vi "FPGA Main Image Processing.vi"(9 "?":T1) -> ()   [LabVIEW 2025]
doc: "The myRIO v1.1 FPGA Shipping Personality. This personality contains support for:\n- 2 Analog Input Interrupt channel\n- 4 Digital Input Interrupt channel\n- 1 Timer\n- 1 Accelerometer\n- 1 Button\n- 4 LED\n- 10 Analog Input channels with 1 Sample\n- 6 Analog Output channels with 1 Sample\n- 40 Digital I/O channels with 1 Sample\n- 2 I2C channels\n- 4 Encoder channels\n- 6 PWM channels\n- 2 SPI channels"
uses:
  SoC IP Library/Controls/Ocurrences.ctl
  SoC IP Library/Controls/Image Size.ctl
  <vilib>/rvi/Emulation/niFpgaGetClockAttributes.vi
  <vilib>/rvi/Emulation/niFpgaSctlEmulationGetInTimedLoop.vi
  <vilib>/rvi/Emulation/niFpgaEmulationReportErrorSimple.vi
  <vilib>/rvi/Emulation/niFpgaProcessEmulError.vi
  <vilib>/rvi/DataTransferAndStorage/Container/Common/niFpgaContainerGetUniqueNameForEmu.vi
  <vilib>/rvi/DataTransferAndStorage/Container/Common/niFpgaContainerSetEmuInfo.vi
  <vilib>/rvi/eio/common/nirviEmuReportErrorAndStop.vi
  <vilib>/rvi/Memory/Memory_Emulation/nirvimemoryFastEmulation.vi
  <vilib>/rvi/Memory/Memory_Emulation/nirvimemoryEmulation.vi
  <vilib>/rvi/Emulation/niFpgaEmulationIsFPGAContextNoSignature.vi
  <vilib>/rvi/errors/nirviReportUnexpectedCaseInternalError (U32).vi
  <vilib>/eio/utilities/niEioResolveVilibRelativePath.vi
  <vilib>/rvi/interface/RandomDataEmulation/niFpgaRandomDataHandleErrors.vi
  <vilib>/rvi/Emulation/niFpgaCriticalErrorInLSC.vi
  <vilib>/rvi/LocalResourceManager/LocalResourceManager.xnode
  <vilib>/rvi/DataTransferAndStorage/Container/XNode/niFpgaContainer.xnode
  <vilib>/rvi/interface/RandomDataEmulation/nirviRandomDataFpgaReadWriteTemplate.vi
  <vilib>/rvi/FXPMathLib/basic elements/FxpDiscreteDelay/XNode/nifxpmath_DiscreteDelay.xnode
  SoC IP Library/SoC IP Library.lvlib
panel:
  out "Current Colum Process":u8
  out "Current Row Process":u8
  out "Current Colum Write":u8
  out "Current Row Write":u8
  out "Current Colum Read":u8
  out "Current Row Read":u8
  out "Pixel B Write":u16
  out "Pixel A Write":u16
  out "SYS.OCURRENCES.RDY":bool
  out "SYS.IMG_SIZE.RDY":bool
  out "Image size":u32
  out "SYS.RDY":bool
  # "Image Processing"
  # "System"
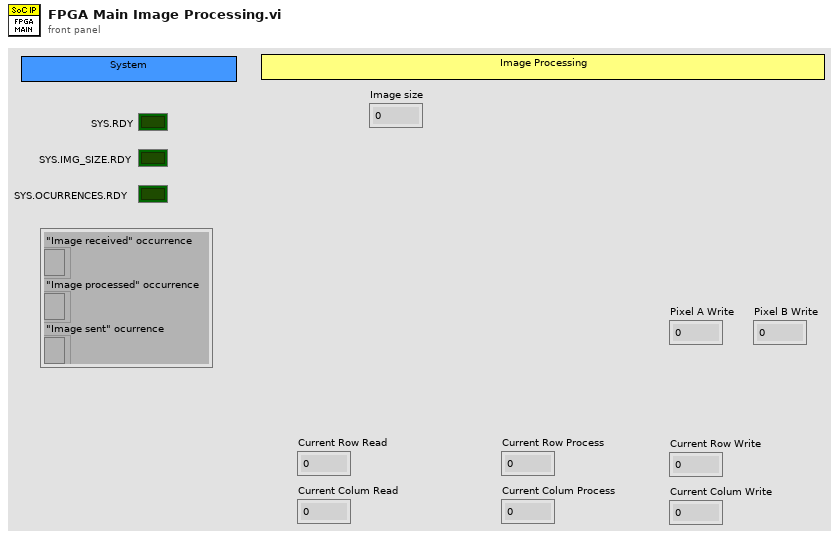
[diagram p1: front panel]
types:
  T1 = typedef "SoC IP Library.lvlib/Ocurrences.ctl" = cluster{"\"Image received\" occurrence":refnum<k4>, "\"Image processed\" occurrence":refnum<k4>, "\"Image sent\" ocurrence":refnum<k4>}
  T2 = typedef "SoC IP Library.lvlib/Image Size.ctl" = cluster{"Rows (X)":u16, "Colums (Y)":u16}
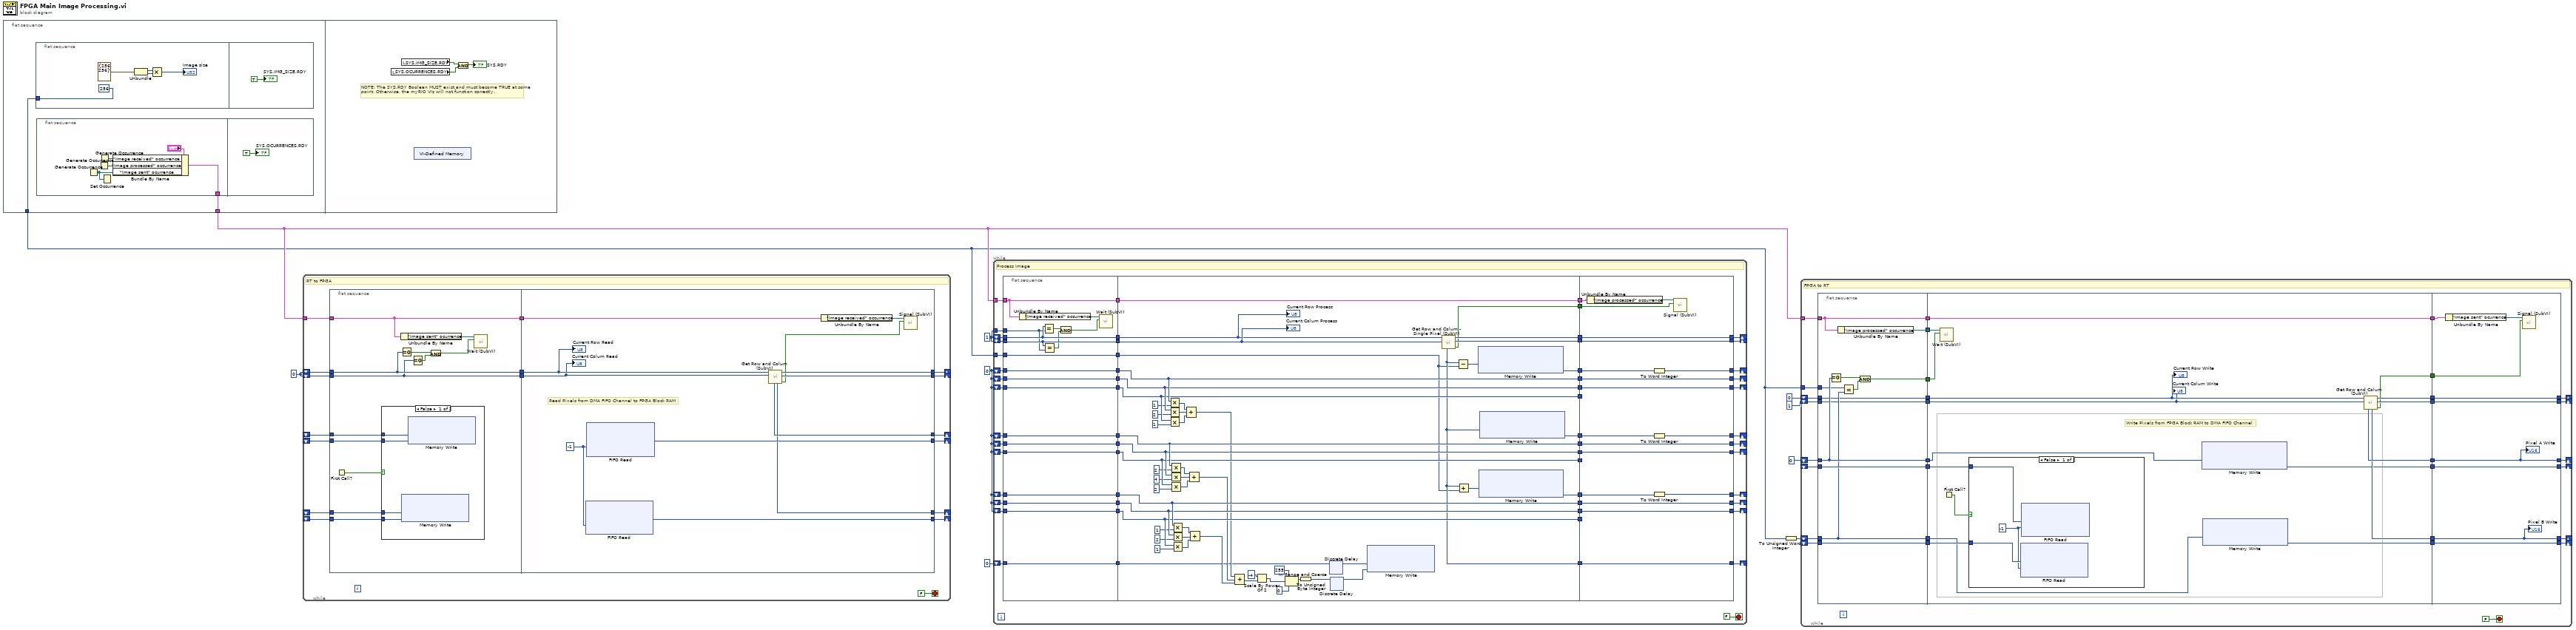
[diagram p0: block diagram]
diagram:
  w2 = i16 0 ("Data")
  w3 = u8 1 ("Row Out")
  w8 = u8 0
  n1 = flat-sequence {
    tunnel: [w12] -> w5
    tunnel: [w11] -> w6
    frame #0 {
      n2 = flat-sequence {
        tunnel: [u32 256 ("Dimension")] -> w12
        frame #0 {
          n3 = Unbundle(T2 {"Rows (X)"=256, "Colums (Y)"=256} ("Image Size")) -> ("Rows (X)"=w21:u16, "Colums (Y)"=w22:u16)
          n4 = Multiply(x=w21, y=w22) -> (x*y=→"Image size":u32)
        }
        frame #1 {
          "SYS.IMG_SIZE.RDY" <- TRUE
        }
      }
      n5 = flat-sequence {
        tunnel: [w13] -> w11
        frame #0 {
          n6 = Generate Occurrence() -> (w14:refnum<k4>)
          n7 = Generate Occurrence() -> (w15:refnum<k4>)
          n8 = Generate Occurrence() -> (w16:refnum<k4>)
          n9 = Set Occurrence(w14) -> ()
          n10 = Bundle By Name(cluster="?", "\"Image received\" occurrence"=w16, "\"Image processed\" occurrence"=w15, "\"Image sent\" ocurrence"=w14) -> (w13:T1)
        }
        frame #1 {
          "SYS.OCURRENCES.RDY" <- TRUE
        }
      }
    }
    frame #1 {
      # "NOTE: The SYS.RDY Boolean MUST exist and must become TRUE at some point. Otherwise, the myRIO VIs will not function correctly."
      n11 = local read "SYS.OCURRENCES.RDY"() -> (w26:bool)
      n12 = local read "SYS.IMG_SIZE.RDY"() -> (w25:bool)
      n13 = xnode "VI-Defined Memory"() -> ()  [unwired: 1 out]
      n14 = And(x=w25, y=w26) -> (x .and. y?=→"SYS.RDY":bool)
    }
  }
  n15 = while {
    shift-right: [w37] -> _
    shift-left: _ -> [w44]
    shift-right: [w31] -> _
    shift-left: _ -> [w43]
    shift-right: [w36] -> _
    shift-left: _ -> [w42]
    shift-right: [w40] -> _
    shift-left: _ -> [w41]
    shift-right: [w39] -> _
    shift-left: w8 -> [w35]
    shift-right: [w38] -> _
    shift-left: w8 -> [w34]
    tunnel: w6 -> [w30]
    stop <- FALSE stop-if-true
    # "RT to FPGA"
    n16 = flat-sequence {
      tunnel: w34 -> [w54]
      tunnel: w35 -> [w55]
      tunnel: w41 -> [w47]
      tunnel: w42 -> [w45]
      tunnel: w43 -> [w48]
      tunnel: w44 -> [w46]
      tunnel: [w55] -> w33
      tunnel: [w54] -> w32
      tunnel: w30 -> [w56]
      tunnel: [w56] -> w29
      tunnel: w33 -> [w68]
      tunnel: w32 -> [w67]
      tunnel: w29 -> [w64]
      tunnel: [w72] -> w31
      tunnel: [w71] -> w40
      tunnel: [w70] -> w39
      tunnel: [w69] -> w38
      tunnel: [w63] -> w37
      tunnel: [w62] -> w36
      frame #0 {
        n17 = First Call?() -> (First Call?: T/F=w49:bool)
        n18 = case shown="False" w49 {
          tunnel: w46 -> [w60 _]
          tunnel: w48 -> [w59 _]
          tunnel: w47 -> [w58 _]
          tunnel: w45 -> [w57 _]
          frame False {
            n19 = xnode ("Memory Write")("Address"=w57, "Data"=w58) -> ()  [unwired: 1 in, 1 out]
            n20 = xnode ("Memory Write")("Address"=w60, "Data"=w59) -> ()  [unwired: 1 in, 1 out]
          }
          frame True {
          }
        }
        n21 = Equal To 0?(x=w55) -> (x = 0?=w52:bool)
        n22 = Unbundle By Name(w56) -> ("\"Image sent\" ocurrence"=w51:refnum<k4>)
        n23 = Equal To 0?(x=w54) -> (x = 0?=w50:bool)
        n24 = And(x=w52, y=w50) -> (x .and. y?=w53:bool)
        n25 = call "Wait (SubVI).vi"("Wait? (T)"=w53, "Occurrence in"=w51) -> ()  [unwired: 10 in]
      }
      frame #1 {
        w65 = -1 ("Timeout")
        # "Read Pixels from DMA FIFO Channel to FPGA Block RAM"
        n26 = xnode ("FIFO Read")("Timeout"=w65) -> ("Element"=w71:u8)  [unwired: 1 in, 2 out]
        n27 = xnode ("FIFO Read")("Timeout"=w65) -> ("Element"=w72:u8)  [unwired: 1 in, 2 out]
        n28 = call "Get Row and Colum (SubVI).vi"("Colum In"=w67, "Row In"=w68) -> ("Last Pixel?"=w66:bool, "Colum Out"=w69:u8, "Row Out"=w70:u8, "Pixel B"=w62:u16, "Pixel A"=w63:u16)  [unwired: 5 in]
        n29 = Unbundle By Name(w64) -> ("\"Image received\" occurrence"=w61:refnum<k4>)
        n30 = call "Signal (SubVI).vi"("Set? (T)"=w66, "Occurrence in"=w61) -> ()  [unwired: 10 in]
        "Current Row Read" <- w68
        "Current Colum Read" <- w67
      }
    }
  }
  n31 = while {
    tunnel: w6 -> [w130]
    shift-right: [w126] -> _
    shift-left: w2 -> [w124]
    shift-right: [w122] -> _
    shift-left: w2 -> [w121]
    shift-right: [w118] -> _
    shift-left: w2 -> [w116]
    shift-right: [w113] -> _
    shift-left: w2 -> [w111]
    shift-right: [w109] -> _
    shift-left: w2 -> [w107]
    shift-right: [w105] -> _
    shift-left: w2 -> [w103]
    shift-right: [w100] -> _
    shift-left: w2 -> [w99]
    shift-right: [w96] -> _
    shift-left: w2 -> [w95]
    shift-right: [w92] -> _
    shift-left: w2 -> [w90]
    shift-right: [w87] -> _
    shift-left: w3 -> [w82]
    shift-right: [w85] -> _
    shift-left: w3 -> [w83]
    tunnel: w5 -> [w80]
    shift-right: [w76] -> _
    shift-left: u32 0 ("Pixel") -> [w78]
    tunnel: w3 -> [w74]
    stop <- FALSE stop-if-true
    # "Process Image"
    n32 = flat-sequence {
      tunnel: w130 -> [w149]
      tunnel: [w149] -> w128
      tunnel: [w148] -> w125
      tunnel: w124 -> [w148]
      tunnel: w121 -> [w147]
      tunnel: [w147] -> w120
      tunnel: [w146] -> w117
      tunnel: w116 -> [w146]
      tunnel: [w145] -> w112
      tunnel: w111 -> [w145]
      tunnel: [w144] -> w108
      tunnel: w107 -> [w144]
      tunnel: [w143] -> w104
      tunnel: w103 -> [w143]
      tunnel: w99 -> [w142]
      tunnel: [w142] -> w98
      tunnel: w95 -> [w141]
      tunnel: [w141] -> w94
      tunnel: [w140] -> w91
      tunnel: w90 -> [w140]
      tunnel: [w137] -> w84
      tunnel: w83 -> [w137]
      tunnel: w82 -> [w136]
      tunnel: [w136] -> w81
      tunnel: w80 -> [w139]
      tunnel: [w139] -> w79
      tunnel: w78 -> [w138]
      tunnel: [w138] -> w77
      tunnel: w74 -> [w135]
      tunnel: [w203] -> w129
      tunnel: w128 -> [w203]
      tunnel: [w202] -> w127
      tunnel: w125 -> [w199]
      tunnel: [w199] -> w123
      tunnel: w120 -> [w198]
      tunnel: [w198] -> w119
      tunnel: w117 -> [w197]
      tunnel: [w197] -> w115
      tunnel: [w201] -> w114
      tunnel: w112 -> [w196]
      tunnel: [w196] -> w110
      tunnel: w108 -> [w195]
      tunnel: [w195] -> w106
      tunnel: w104 -> [w194]
      tunnel: [w194] -> w102
      tunnel: [w200] -> w101
      tunnel: w98 -> [w193]
      tunnel: [w193] -> w97
      tunnel: w94 -> [w192]
      tunnel: [w192] -> w93
      tunnel: w91 -> [w191]
      tunnel: [w191] -> w89
      tunnel: [w169] -> w88
      tunnel: [w168] -> w86
      tunnel: w84 -> [w161]
      tunnel: w81 -> [w162]
      tunnel: w79 -> [w163]
      tunnel: w77 -> [w152]
      tunnel: [w165] -> w75
      tunnel: [w160] -> w73
      tunnel: w129 -> [w221]
      tunnel: w127 -> [w219]
      tunnel: [w207] -> w126
      tunnel: w123 -> [w218]
      tunnel: [w218] -> w122
      tunnel: w119 -> [w217]
      tunnel: [w217] -> w118
      tunnel: w115 -> [_]
      tunnel: w114 -> [w216]
      tunnel: [w206] -> w113
      tunnel: w110 -> [w215]
      tunnel: [w215] -> w109
      tunnel: w106 -> [w214]
      tunnel: [w214] -> w105
      tunnel: w102 -> [_]
      tunnel: w101 -> [w205]
      tunnel: [w204] -> w100
      tunnel: w97 -> [w213]
      tunnel: [w213] -> w96
      tunnel: w93 -> [w212]
      tunnel: [w212] -> w92
      tunnel: w89 -> [_]
      tunnel: [w211] -> w87
      tunnel: w88 -> [w211]
      tunnel: w86 -> [w210]
      tunnel: [w210] -> w85
      tunnel: [w209] -> w76
      tunnel: w75 -> [w209]
      tunnel: w73 -> [w208]
      frame #0 {
        n33 = Unbundle By Name(w149) -> ("\"Image received\" occurrence"=w150:refnum<k4>)
        n34 = Equal?(x=w137, y=w135) -> (x = y?=w134:bool)
        n35 = Equal?(x=w136, y=w135) -> (x = y?=w133:bool)
        n36 = And(x=w134, y=w133) -> (x .and. y?=w132:bool)
        n37 = call "Wait (SubVI).vi"("Wait? (T)"=w132, "Occurrence in"=w150) -> ()  [unwired: 10 in]
      }
      frame #1 {
        n38 = Multiply(x=w199, y=i16 1) -> (x*y=w185:i16)
        n39 = Multiply(x=w198, y=i16 2) -> (x*y=w187:i16)
        n40 = Multiply(x=w197, y=i16 1) -> (x*y=w186:i16)
        n41 = Multiply(x=w196, y=i16 2) -> (x*y=w184:i16)
        n42 = Multiply(x=w195, y=i16 4) -> (x*y=w183:i16)
        n43 = Multiply(x=w194, y=i16 2) -> (x*y=w182:i16)
        n44 = Multiply(x=w193, y=i16 1) -> (x*y=w190:i16)
        n45 = Multiply(x=w192, y=i16 2) -> (x*y=w189:i16)
        n46 = Multiply(x=w191, y=i16 1) -> (x*y=w188:i16)
        n47 = Compound Arithmetic op=ADD(w185, w187, w186) -> (w181:i16)
        n48 = Compound Arithmetic op=ADD(w184, w183, w182) -> (w180:i16)
        n49 = Compound Arithmetic op=ADD(w190, w189, w188) -> (w179:i16)
        n50 = Compound Arithmetic op=ADD(w181, w180, w179) -> (w157:i16)
        n51 = Scale By Power Of 2(n=i16 -4, x=w157) -> (x*2^n=w155:i16)
        n52 = In Range and Coerce(upper limit=i16 255, x=w155, lower limit=i16 0) -> (coerced(x)=w158:i16)  [unwired: 1 out]
        n53 = To Unsigned Byte Integer(number=w158) -> (unsigned 8bit integer=w154:u8)
        n54 = xnode ("Discrete Delay")("D"=w152) -> ("Q"=w151:u32)
        n55 = xnode ("Discrete Delay")("D"=w154) -> ("Q"=w153:u8)
        n56 = xnode ("Memory Write")("Address"=w151, "Data"=w153) -> ()  [unwired: 1 in, 1 out]
        n57 = call "Get Row and Colum - Single Pixel (SubVI).vi"("Colum In"=w162, "Row In"=w161) -> ("Last Pixel?"=w160:bool, "Colum Out"=w169:u8, "Row Out"=w168:u8, "Pixel"=w165:u16)  [unwired: 6 in]
        n58 = Subtract(x=w165, y=w163) -> (x-y=w166:u32)
        n59 = Add(x=w165, y=w163) -> (x+y=w167:u32)
        n60 = xnode ("Memory Write")("Address"=w166) -> ("Data"=w202:u8)  [unwired: 1 in, 1 out]
        n61 = xnode ("Memory Write")("Address"=w167) -> ("Data"=w200:u8)  [unwired: 1 in, 1 out]
        n62 = xnode ("Memory Write")("Address"=w165) -> ("Data"=w201:u8)  [unwired: 1 in, 1 out]
        "Current Row Process" <- w161
        "Current Colum Process" <- w162
      }
      frame #2 {
        n63 = Unbundle By Name(w221) -> ("\"Image processed\" occurrence"=w220:refnum<k4>)
        n64 = To Word Integer(number=w205) -> (16bit integer=w204:i16)
        n65 = To Word Integer(number=w219) -> (16bit integer=w207:i16)
        n66 = To Word Integer(number=w216) -> (16bit integer=w206:i16)
        n67 = call "Signal (SubVI).vi"("Set? (T)"=w208, "Occurrence in"=w220) -> ()  [unwired: 10 in]
      }
    }
  }
  n68 = To Unsigned Word Integer(number=w5) -> (unsigned 16bit integer=w1:u16)
  n69 = while {
    shift-right: [w249] -> _
    shift-left: u16 0 -> [w253]
    shift-right: [w248] -> _
    shift-left: w1 -> [w252]
    shift-right: [w251] -> _
    shift-left: u8 0 -> [w247]
    shift-right: [w250] -> _
    shift-left: u8 1 ("Colum Out") -> [w246]
    shift-right: [w237] -> _
    shift-left: _ -> [w233]
    shift-right: [w235] -> _
    shift-left: _ -> [w231]
    tunnel: w5 -> [w227]
    tunnel: w6 -> [w226]
    stop <- FALSE stop-if-true
    # "FPGA to RT"
    n70 = flat-sequence {
      tunnel: w246 -> [w257]
      tunnel: w247 -> [w258]
      tunnel: w252 -> [w260]
      tunnel: w253 -> [w261]
      tunnel: [w261] -> w245
      tunnel: [w260] -> w244
      tunnel: [w263] -> w234
      tunnel: w233 -> [w263]
      tunnel: [w262] -> w232
      tunnel: w231 -> [w262]
      tunnel: [w259] -> w230
      tunnel: [w258] -> w229
      tunnel: [w257] -> w228
      tunnel: w227 -> [w256]
      tunnel: w226 -> [w255]
      tunnel: [w255] -> w225
      tunnel: [w254] -> w223
      tunnel: w245 -> [w272]
      tunnel: w244 -> [w271]
      tunnel: [w282] -> w243
      tunnel: [w281] -> w242
      tunnel: [w280] -> w241
      tunnel: [w279] -> w240
      tunnel: [w278] -> w239
      tunnel: [w277] -> w238
      tunnel: [w276] -> w236
      tunnel: w234 -> [w275]
      tunnel: w232 -> [w274]
      tunnel: w230 -> [w268]
      tunnel: w229 -> [w270]
      tunnel: w228 -> [w269]
      tunnel: w225 -> [w267]
      tunnel: [w267] -> w224
      tunnel: w223 -> [w266]
      tunnel: [w291] -> w248
      tunnel: [w292] -> w249
      tunnel: [w293] -> w250
      tunnel: [w294] -> w251
      tunnel: w243 -> [w294]
      tunnel: w242 -> [w293]
      tunnel: w241 -> [w292]
      tunnel: w240 -> [w291]
      tunnel: w239 -> [w288]
      tunnel: [w290] -> w237
      tunnel: w238 -> [w290]
      tunnel: [w289] -> w235
      tunnel: w236 -> [w289]
      tunnel: w224 -> [w287]
      frame #0 {
        n71 = Equal To 0?(x=w261) -> (x = 0?=w264:bool)
        n72 = Unbundle By Name(w255) -> ("\"Image processed\" occurrence"=w254:refnum<k4>)
        n73 = Equal?(x=w256, y=w260) -> (x = y?=w265:bool)
        n74 = And(x=w264, y=w265) -> (x .and. y?=w259:bool)
      }
      frame #1 {
        # "Write Pixels from FPGA Block RAM to DMA FIFO Channel"
        n75 = call "Wait (SubVI).vi"("Wait? (T)"=w268, "Occurrence in"=w266) -> ()  [unwired: 10 in]
        n76 = First Call?() -> (First Call?: T/F=w273:bool)
        n77 = case shown="False" w273 {
          tunnel: w275 -> [w285 _]
          tunnel: w274 -> [w284 _]
          frame False {
            w283 = -1 ("Timeout")
            n78 = xnode ("FIFO Read")("Element"=w284, "Timeout"=w283) -> ()  [unwired: 1 in, 2 out]
            n79 = xnode ("FIFO Read")("Element"=w285, "Timeout"=w283) -> ()  [unwired: 1 in, 2 out]
          }
          frame True {
          }
        }
        n80 = xnode ("Memory Write")("Address"=w272) -> ("Data"=w277:u8)  [unwired: 1 in, 1 out]
        n81 = xnode ("Memory Write")("Address"=w271) -> ("Data"=w276:u8)  [unwired: 1 in, 1 out]
        n82 = call "Get Row and Colum (SubVI).vi"("Colum In"=w269, "Row In"=w270) -> ("Last Pixel?"=w278:bool, "Colum Out"=w281:u8, "Row Out"=w282:u8, "Pixel B"=w279:u16, "Pixel A"=w280:u16)  [unwired: 5 in]
        "Current Row Write" <- w270
        "Current Colum Write" <- w269
      }
      frame #2 {
        n83 = Unbundle By Name(w287) -> ("\"Image sent\" ocurrence"=w286:refnum<k4>)
        n84 = call "Signal (SubVI).vi"("Set? (T)"=w288, "Occurrence in"=w286) -> ()  [unwired: 10 in]
        "Pixel A Write" <- w292
        "Pixel B Write" <- w291
      }
    }
  }
